vi "New Message.vi"(8 "error in (no error)":errorcluster, 10 "New Message":string, 11 "BuildWorker in":refnum<class "BuildWorker.lvclass">) -> (0 "error out":errorcluster, 3 "BuildWorker out":refnum<class "BuildWorker.lvclass">)   [LabVIEW 2017, in "BuildWorker.lvlib" / "BuildWorker.lvclass"]
uses:
  BuildWorker.lvclass
  <vilib>/ActorFramework/Actor/Actor.lvclass
  Classes/Message Interface/Command/Command.lvclass
  Volumes/Data/Users/benji667/Git/BuildFarm/src/LabVIEW/vi.lib/BenjaminR/Build Farm/Actors/Framework/Actor wUI/Actor wUI.lvclass
  Applications/National Instruments/LabVIEW 2017 64-bit/vi.lib/ActorFramework/Actor/Actor.lvclass
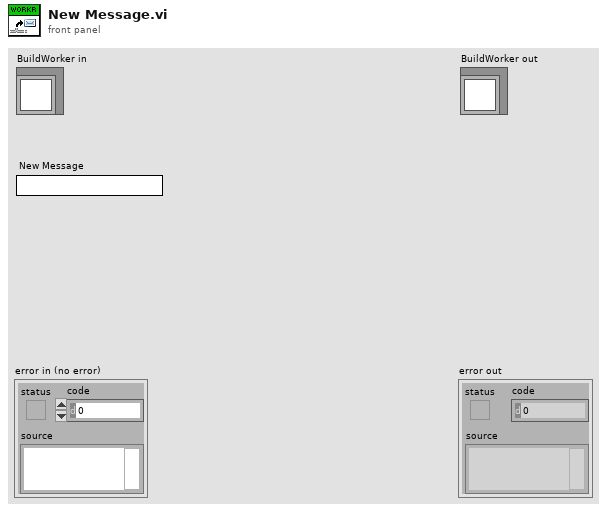
[diagram p1: front panel]
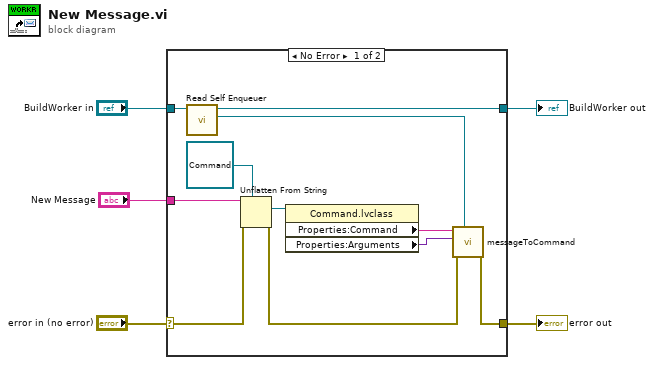
[diagram p0: block diagram]
diagram:
  n1 = case shown="No Error" "error in (no error)" {
    selector: "error in (no error)" -> [w14 w17]
    tunnel: [w11 w17] -> w4
    tunnel: [w15 w16] -> w2
    tunnel: "BuildWorker in" -> [w15 w16]
    tunnel: "New Message" -> [w9 _]
    frame No Error {
      n2 = call <vilib>:"Read Self Enqueuer.vi"("Actor"=w15) -> ("Self Enqueuer"=w13:refnum<class "Message Enqueuer.lvclass">)  [unwired: 10 in]
      n3 = Unflatten From String(type=refnum<class "Command.lvclass"> refnum ("Command.lvclass"), binary string=w9, error in (no error)=w14) -> (value=w8:refnum<class "Command.lvclass">, error out=w12:errorcluster)  [unwired: 2 in, 1 out]
      n4 = property class="Command.lvclass"(reference=w8) -> ("Properties:Command"=w7:string, "Properties:Arguments"=w6:variant)  [unwired: 1 in, 2 out]
      n5 = call "messageToCommand.vi"("Self Enqueuer"=w13, "error in (no error)"=w12, "Arguments"=w6, "Command"=w7) -> ("error out"=w11:errorcluster)  [unwired: 7 in]
    }
    frame Error {
    }
  }
  "error out" <- w4
  "BuildWorker out" <- w2
